vi "油压显示.vi"() -> ()   [LabVIEW 2013]
panel:
  out "油压显示":bool
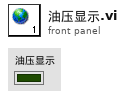
[diagram p1: front panel]
diagram:
